vi "ReadDialogStatus.vi"(8 "error in (no error)":errorcluster, 9 "BuildType":T1 items=["simple", "Dialog", "PVUpdate", "Dialog&PV", "Asynch", "AsynchDial", "Ack"], 10 "Configure Dialog?":bool, 11 "ClassReference":refnum<vi>) -> (0 "error out":errorcluster, 2 "ModifyDialog":bool, 3 "reference out":refnum<vi>)   [LabVIEW 2016, in "CS++Actor.lvlib" / "CS++Actor.lvclass"]
uses:
  CS++Actor.lvclass
  CSPP_MessageMakerMain/BuildType.ctl
  CSPP_Message/MessageStatus.ctl
  CSPP_MessageMakerMain/CS++MessageMakerMain.lvclass
  CSPP_Message/CS++Message.lvclass
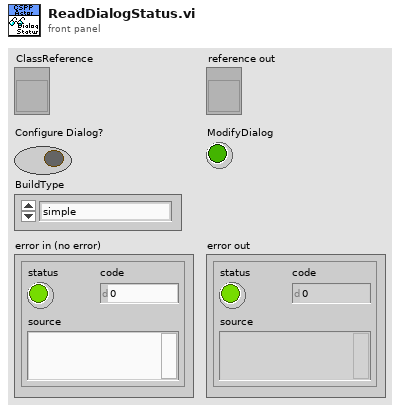
[diagram p1: front panel]
types:
  T1 = typedef "CS++MessageMakerMain.lvlib/CS++MessageMakerMain.lvclass/BuildType.ctl" = u16
  T2 = typedef "CS++Message.lvlib/CS++Message.lvclass/MessageStatus.ctl" = u16
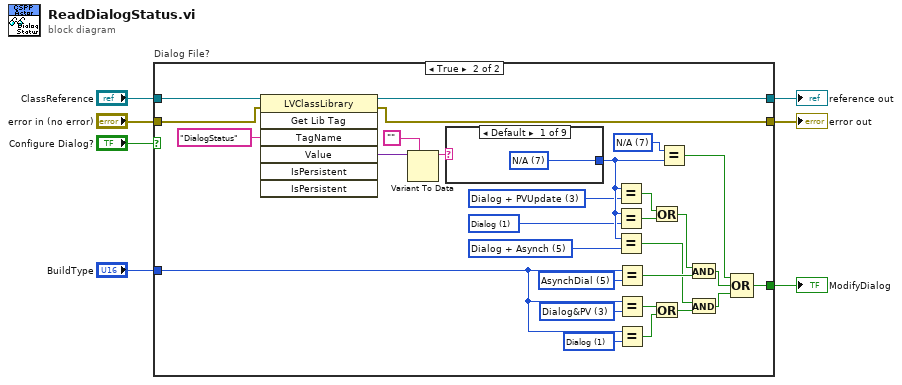
[diagram p0: block diagram]
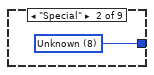
[diagram p3: hidden frame]
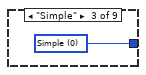
[diagram p4: hidden frame]
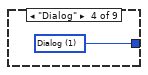
[diagram p5: hidden frame]
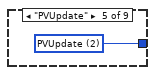
[diagram p6: hidden frame]
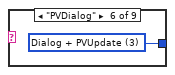
[diagram p7: hidden frame]
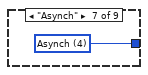
[diagram p8: hidden frame]
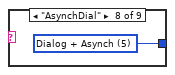
[diagram p9: hidden frame]
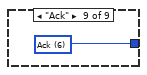
[diagram p10: hidden frame]
diagram:
  n1 = case "Dialog File?" shown="True" "Configure Dialog?" {
    tunnel: "ClassReference" -> [w9 w37]
    tunnel: "error in (no error)" -> [w8 w36]
    tunnel: [w8 w35] -> w4
    tunnel: [w9 w34] -> w3
    tunnel: "BuildType" -> [_ w19]
    tunnel: [_ w20] -> w1
    frame False {
    }
    frame True {
      w10 = T1 1 items=["simple", "Dialog", "PVUpdate", "Dialog&PV", "Asynch", "AsynchDial", "Ack"] ("BuildType")
      w11 = T1 3 items=["simple", "Dialog", "PVUpdate", "Dialog&PV", "Asynch", "AsynchDial", "Ack"] ("BuildType")
      w12 = T1 5 items=["simple", "Dialog", "PVUpdate", "Dialog&PV", "Asynch", "AsynchDial", "Ack"] ("BuildType")
      w13 = T2 5 items=["Simple", "Dialog", "PVUpdate", "Dialog + PVUpdate", "Asynch", "Dialog + Asynch", "Ack", "N/A", "Unknown"] ("Message Status")
      w14 = T2 1 items=["Simple", "Dialog", "PVUpdate", "Dialog + PVUpdate", "Asynch", "Dialog + Asynch", "Ack", "N/A", "Unknown"] ("Message Status")
      w15 = T2 3 items=["Simple", "Dialog", "PVUpdate", "Dialog + PVUpdate", "Asynch", "Dialog + Asynch", "Ack", "N/A", "Unknown"] ("Message Status")
      w16 = T2 7 items=["Simple", "Dialog", "PVUpdate", "Dialog + PVUpdate", "Asynch", "Dialog + Asynch", "Ack", "N/A", "Unknown"] ("Message Status")
      n2 = invoke class="LVClassLibrary" method="Get Lib Tag"(reference=w37, error in=w36, "TagName"="DialogStatus" ("Tag Name")) -> (reference out=w34:refnum<vi>, error out=w35:errorcluster, "Value"=w32:variant)  [unwired: 4 in, 4 out]
      n3 = Variant To Data(type="", Variant=w32) -> (data=w31:string)  [unwired: 1 in, 1 out]
      n4 = case shown="Default" w31 {
        tunnel: [w39 w40 w41 w42 w43 w44 w45 w46 w47] -> w18
        frame Default {
          w39 = T2 7 items=["Simple", "Dialog", "PVUpdate", "Dialog + PVUpdate", "Asynch", "Dialog + Asynch", "Ack", "N/A", "Unknown"] ("Message Status")
        }
        frame "Special" {
          w40 = T2 8 items=["Simple", "Dialog", "PVUpdate", "Dialog + PVUpdate", "Asynch", "Dialog + Asynch", "Ack", "N/A", "Unknown"] ("Message Status")
        }
        frame "Simple" {
          w41 = T2 0 items=["Simple", "Dialog", "PVUpdate", "Dialog + PVUpdate", "Asynch", "Dialog + Asynch", "Ack", "N/A", "Unknown"] ("Message Status")
        }
        frame "Dialog" {
          w42 = T2 1 items=["Simple", "Dialog", "PVUpdate", "Dialog + PVUpdate", "Asynch", "Dialog + Asynch", "Ack", "N/A", "Unknown"] ("Message Status")
        }
        frame "PVUpdate" {
          w43 = T2 2 items=["Simple", "Dialog", "PVUpdate", "Dialog + PVUpdate", "Asynch", "Dialog + Asynch", "Ack", "N/A", "Unknown"] ("Message Status")
        }
        frame "PVDialog" {
          w44 = T2 3 items=["Simple", "Dialog", "PVUpdate", "Dialog + PVUpdate", "Asynch", "Dialog + Asynch", "Ack", "N/A", "Unknown"] ("Message Status")
        }
        frame "Asynch" {
          w45 = T2 4 items=["Simple", "Dialog", "PVUpdate", "Dialog + PVUpdate", "Asynch", "Dialog + Asynch", "Ack", "N/A", "Unknown"] ("Message Status")
        }
        frame "AsynchDial" {
          w46 = T2 5 items=["Simple", "Dialog", "PVUpdate", "Dialog + PVUpdate", "Asynch", "Dialog + Asynch", "Ack", "N/A", "Unknown"] ("Message Status")
        }
        frame "Ack" {
          w47 = T2 6 items=["Simple", "Dialog", "PVUpdate", "Dialog + PVUpdate", "Asynch", "Dialog + Asynch", "Ack", "N/A", "Unknown"] ("Message Status")
        }
      }
      n5 = Equal?(x=w18, y=w15) -> (x = y?=w29:bool)
      n6 = Equal?(x=w18, y=w14) -> (x = y?=w28:bool)
      n7 = Equal?(x=w18, y=w13) -> (x = y?=w23:bool)
      n8 = Equal?(x=w19, y=w12) -> (x = y?=w30:bool)
      n9 = Equal?(x=w19, y=w11) -> (x = y?=w26:bool)
      n10 = Equal?(x=w19, y=w10) -> (x = y?=w25:bool)
      n11 = Or(x=w29, y=w28) -> (x .or. y?=w27:bool)
      n12 = Or(x=w26, y=w25) -> (x .or. y?=w24:bool)
      n13 = Equal?(x=w16, y=w18) -> (x = y?=w17:bool)
      n14 = And(x=w27, y=w30) -> (x .and. y?=w22:bool)
      n15 = And(x=w23, y=w24) -> (x .and. y?=w21:bool)
      n16 = Compound Arithmetic op=OR(w17, w22, w21) -> (w20:bool)
    }
  }
  "error out" <- w4
  "reference out" <- w3
  "ModifyDialog" <- w1
